vi "microstep_resolution.vi"(8 "error in (no error)":errorcluster, 10 "number":i32, 11 "VISA in":refnum<visa-resource-name>) -> (0 "error out":errorcluster, 3 "VISA out":refnum<visa-resource-name>)   [LabVIEW 2019]
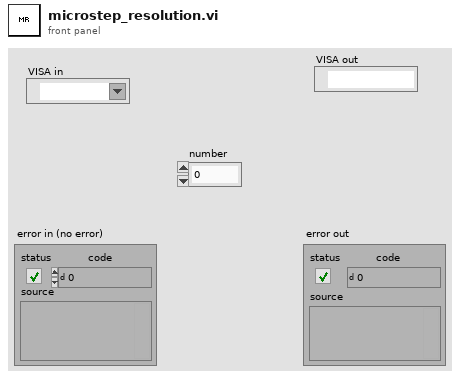
[diagram p1: front panel]
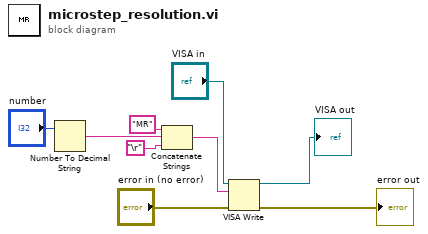
[diagram p0: block diagram]
diagram:
  n1 = Number To Decimal String(number="number") -> (decimal integer string=w2:string)  [unwired: 1 in]
  n2 = Concatenate Strings("MR", w2, "\r") -> (w9:string)
  n3 = VISA Write(VISA resource name="VISA in", write buffer=w9, error in (no error)="error in (no error)") -> (VISA resource name out=→"VISA out":refnum<visa-resource-name>, error out=→"error out":errorcluster)  [unwired: 1 out]
